vi "init.vi"(8 "error in (no error)":errorcluster, 10 "Tests To Execute":T1[](array[typedef]), 11 "TestSeries in":refnum<class "TestSeries.lvclass">) -> (0 "error out":errorcluster, 3 "TestSeries out":refnum<class "TestSeries.lvclass">)   [LabVIEW 2015, in "TestSeries.lvclass"]
uses:
  TestSeries.lvclass
  Typedefs/TestScenarioTypes.ctl
  TestSeries.lvclass/TestSeries.ctl
  Typedefs/ILCBTTypedefs.lvlib
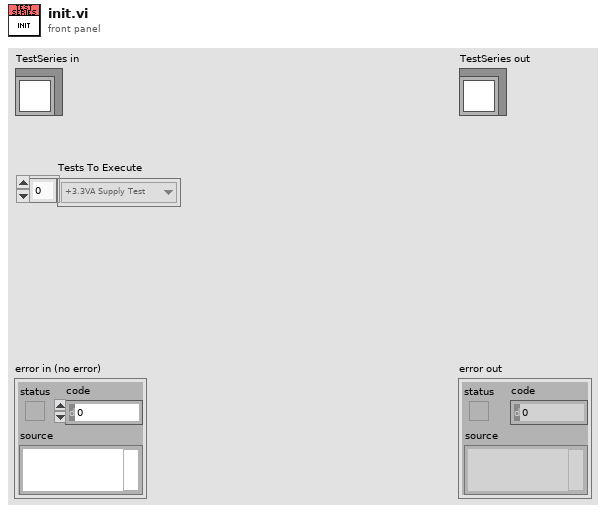
[diagram p1: front panel]
types:
  T1 = typedef "ILCBTTypedefs.lvlib/TestScenarioTypes.ctl" = enum16{"+3.3VA Supply Test", "+3.3VD Supply Test", "+5VA Supply Test", "+5VD Supply Test", "Unique ID Test", "TEDS Status Test", "LIMSW1_TTL Low Test", "LIMSW1_TTL High Test", "LIMSW2_TTL Low Test", "LIMSW2_TTL High Test", "Tachometer Low Test", "Tachometer High Test", "SSR_TTL Low Test", "SSR_TTL High Test", "SM_GPI Low Test", "SM_GPI High Test", "CW Motion Without Limit Test", "CW Motion With Limit Test", "CW Motion With Both Limits Test", "CW Motion on CCW Limit Test", "CCW Motion Without Limit Test", "CCW Motion With Limit Test", "CCW Motion With Both Limits Test", "CCW Motion on CW Limit Test", "RS232-TXD Low Test", "RS232-TXD High Test", "RS232-RTS Low Test", "RS232-RTS High Test", "RS232-RXD Low Test", "RS232-RXD High Test", "RS232-CTS Low Test", "RS232-CTS High Test", "Out_SS Low Test", "Out_SS High Test", "Out_SDI Low Test", "Out_SDI High Test", "Out_SCLK Low Test", "Out_SCLK High Test", "Reset Low Test", "Reset High Test", "1 Channel ADC Test", "3 Channel ADC Test", "5 Channel ADC Test", "Vref Test", "ROT Test", "DAC1 Test", "DAC2 Test", "DAC3 Test", "DAC4 Test", "BIAS Test", "EXC1 Test", "EXC2 Test", "EXC3 Test", "EXC4 Test"}
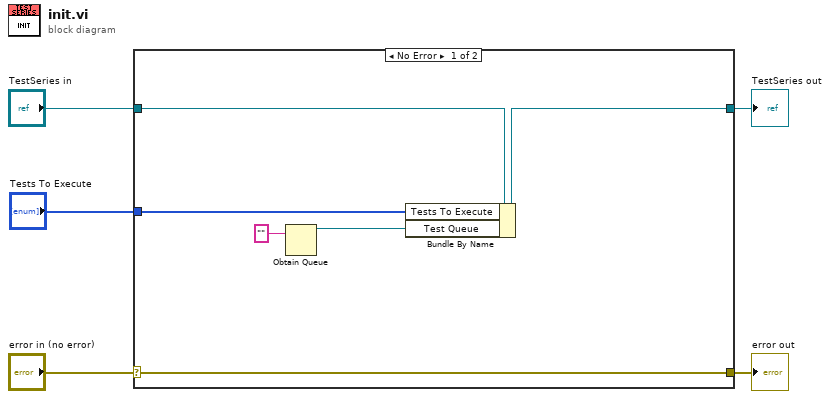
[diagram p0: block diagram]
diagram:
  n1 = case shown="No Error" "error in (no error)" {
    selector: "error in (no error)" -> [w11 w13]
    tunnel: [w11 w13] -> w4
    tunnel: [w8 w12] -> w2
    tunnel: "TestSeries in" -> [w9 w12]
    tunnel: "Tests To Execute" -> [w10 _]
    frame No Error {
      n2 = Obtain Queue(element data type="") -> (queue out=w6:refnum<queue>)  [unwired: 4 in, 2 out]
      n3 = Bundle By Name(cluster=w9, "Tests To Execute"=w10, "Test Queue"=w6) -> (w8:refnum<class "TestSeries.lvclass">)
    }
    frame Error {
    }
  }
  "error out" <- w4
  "TestSeries out" <- w2
